vi "Parse NavData.vi"(11 "NavData Port":refnum<k16>) -> (1 "NavData":T1, 3 "NavData Port":refnum<k16>)   [LabVIEW 2011]
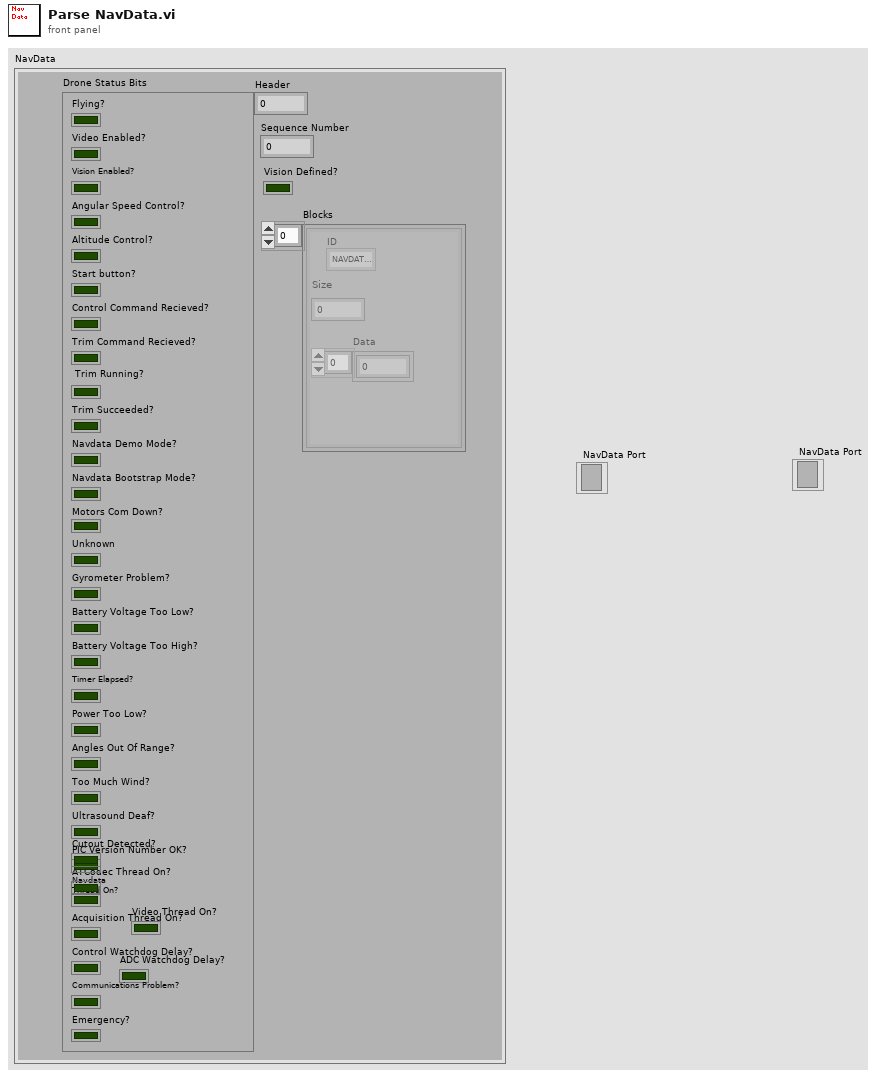
[diagram p1: front panel]
types:
  T1 = cluster{"Drone Status Bits":cluster{"Flying?":bool, "Video Enabled?":bool, "Vision Enabled?":bool, "Angular Speed Control?":bool, "Altitude Control?":bool, "Start button?":bool, "Control Command Recieved?":bool, "Trim Command Recieved?":bool, "Trim Running?":bool, "Trim Succeeded?":bool, "Navdata Demo Mode?":bool, "Navdata Bootstrap Mode?":bool, "Motors Com Down?":bool, "Unknown":bool, "Gyrometer Problem?":bool, "Battery Voltage Too Low?":bool, "Battery Voltage Too High?":bool, "Timer Elapsed?":bool, "Power Too Low?":bool, "Angles Out Of Range?":bool, "Too Much Wind?":bool, "Ultrasound Deaf?":bool, "Cutout Detected?":bool, "PIC Version Number OK?":bool, "ATCodec Thread On?":bool, "Navdata Thread On?":bool, "Video Thread On?":bool, "Acquisition Thread On?":bool, "Control Watchdog Delay?":bool, "ADC Watchdog Delay?":bool, "Communications Problem?":bool, "Emergency?":bool}, "Header":u32, "Sequence Number":u32, "Vision Defined?":bool, "Blocks":cluster{"Size":u16, "Data":u8[], "ID":enum16{"NAVDATA_DEMO", "NAVDATA_TIME", "NAVDATA_RAW_MEASURES", "NAVDATA_PHYS_MEASURES", "NAVDATA_GYROS_OFFSETS", "NAVDATA_EULER_ANGLES", "NAVDATA_REFERENCES", "NAVDATA_TRIMS", "NAVDATA_RC_REFERENCES", "NAVDATA_PWM", "NAVDATA_ALTITUDE", "NAVDATA_VISION_RAW", "NAVDATA_VISION_OF", "NAVDATA_VISION", "NAVDATA_VISION_PERF", "NAVDATA_TRACKERS_SEND", "NAVDATA_VISION_DETECT", "NAVDATA_WATCHDOG", "NAVDATA_ADC_DATA_FRAME", "NAVDATA_VIDEO_STREAM", "NAVDATA_GAMES"}}[]}
  T2 = cluster{"Size":u16, "Data":u8[], "ID":enum16{"NAVDATA_DEMO", "NAVDATA_TIME", "NAVDATA_RAW_MEASURES", "NAVDATA_PHYS_MEASURES", "NAVDATA_GYROS_OFFSETS", "NAVDATA_EULER_ANGLES", "NAVDATA_REFERENCES", "NAVDATA_TRIMS", "NAVDATA_RC_REFERENCES", "NAVDATA_PWM", "NAVDATA_ALTITUDE", "NAVDATA_VISION_RAW", "NAVDATA_VISION_OF", "NAVDATA_VISION", "NAVDATA_VISION_PERF", "NAVDATA_TRACKERS_SEND", "NAVDATA_VISION_DETECT", "NAVDATA_WATCHDOG", "NAVDATA_ADC_DATA_FRAME", "NAVDATA_VIDEO_STREAM", "NAVDATA_GAMES"}}[]
  T3 = cluster{"Size":u16, "Data":u8[], "ID":enum16{"NAVDATA_DEMO", "NAVDATA_TIME", "NAVDATA_RAW_MEASURES", "NAVDATA_PHYS_MEASURES", "NAVDATA_GYROS_OFFSETS", "NAVDATA_EULER_ANGLES", "NAVDATA_REFERENCES", "NAVDATA_TRIMS", "NAVDATA_RC_REFERENCES", "NAVDATA_PWM", "NAVDATA_ALTITUDE", "NAVDATA_VISION_RAW", "NAVDATA_VISION_OF", "NAVDATA_VISION", "NAVDATA_VISION_PERF", "NAVDATA_TRACKERS_SEND", "NAVDATA_VISION_DETECT", "NAVDATA_WATCHDOG", "NAVDATA_ADC_DATA_FRAME", "NAVDATA_VIDEO_STREAM", "NAVDATA_GAMES"}}
  T4 = cluster{"Boolean array[0]":bool, "Boolean array[1]":bool, "Boolean array[2]":bool, "Boolean array[3]":bool, "Boolean array[4]":bool, "Boolean array[5]":bool, "Boolean array[6]":bool, "Boolean array[7]":bool, "Boolean array[8]":bool, "Boolean array[9]":bool, "Boolean array[10]":bool, "Boolean array[11]":bool, "Boolean array[12]":bool, "Boolean array[13]":bool, "Boolean array[14]":bool, "Boolean array[15]":bool, "Boolean array[16]":bool, "Boolean array[17]":bool, "Boolean array[18]":bool, "Boolean array[19]":bool, "Boolean array[20]":bool, "Boolean array[21]":bool, "Boolean array[22]":bool, "Boolean array[23]":bool, "Boolean array[24]":bool, "Boolean array[25]":bool, "Boolean array[26]":bool, "Boolean array[27]":bool, "Boolean array[28]":bool, "Boolean array[29]":bool, "Boolean array[30]":bool, "Boolean array[31]":bool}
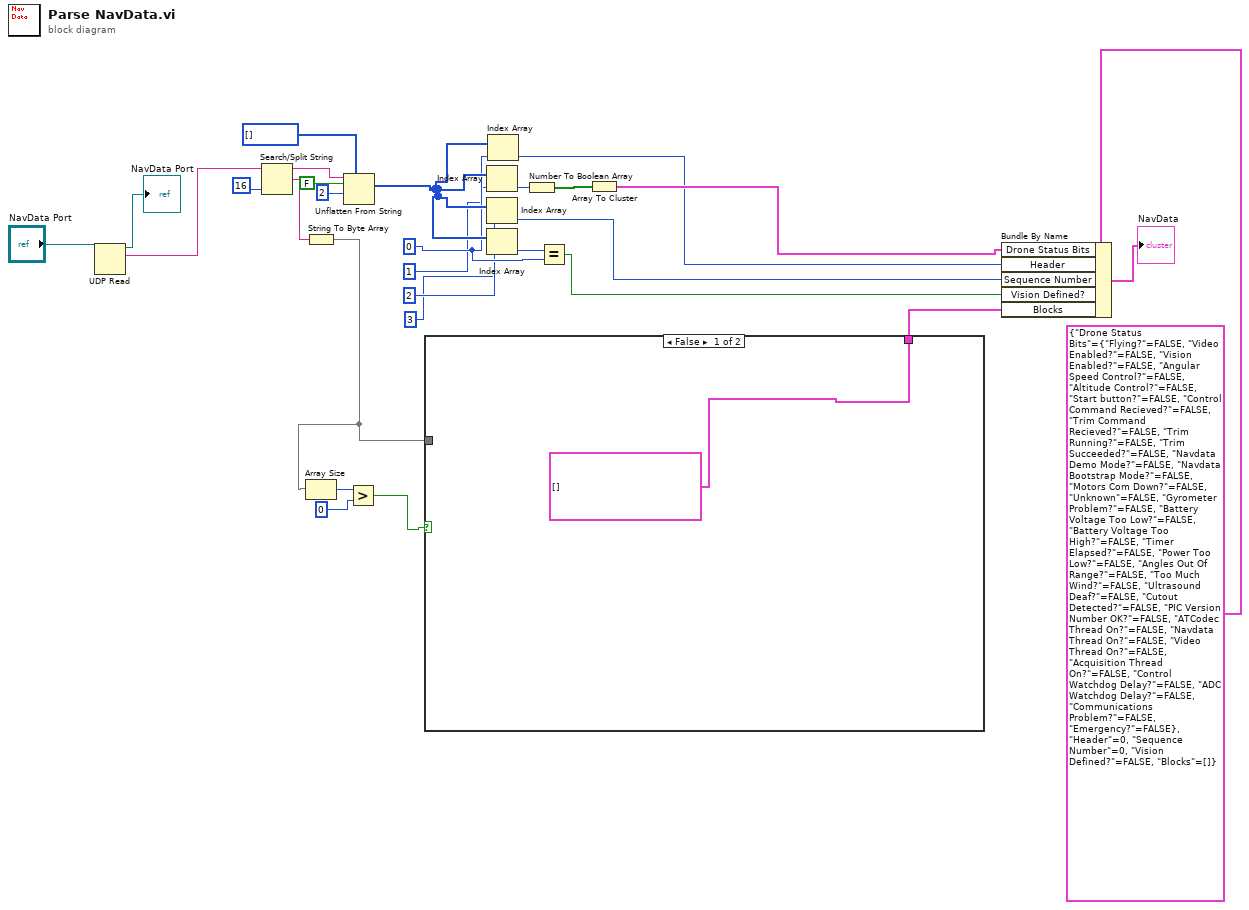
[diagram p0: block diagram]
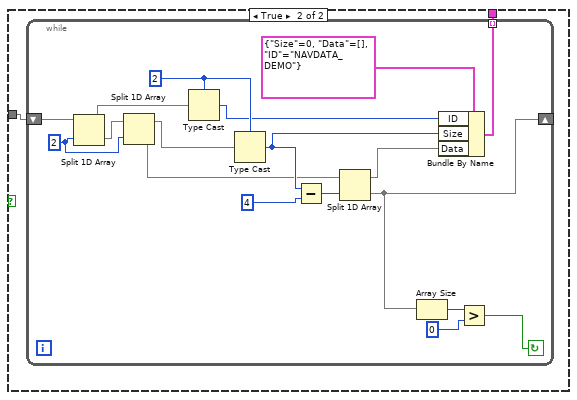
[diagram p2: hidden frame]
diagram:
  w18 = 0
  n1 = UDP Read(connection ID="NavData Port") -> (data out=w2:string, 3:→"NavData Port":refnum<k16>)  [unwired: 3 in, 3 out]
  n2 = Search/Split String(string=w2, offset (0)=16) -> (substring before match=w11:string, match + rest of string=w10:string)  [unwired: 1 in, 1 out]
  n3 = String To Byte Array(string=w10) -> (unsigned byte array=w9:u8[])
  n4 = Array Size(array=w9) -> (size(s)=w8:i32)
  n5 = Unflatten From String(type=u32[] [], binary string=w11, data includes array or string size? (T)=FALSE, byte order (0:big-endian, network order)=u32 2) -> (value=w19:u32[])  [unwired: 1 in, 2 out]
  n6 = Greater?(x=w8, y=0) -> (0:w6:bool)
  n7 = case shown="False" w6 {
    tunnel: w9 -> [_ w31]
    tunnel: [T2 [] ("Blocks") w30] -> w4
    frame False {
    }
    frame True {
      n8 = while {
        shift-right: [w33] -> _
        shift-left: w31 -> [w49]
        tunnel: [w48] -> w30 mode=indexing
        stop <- w34 continue-if-true
        w43 = u16 2
        w46 = 2
        n9 = Split 1D Array(array=w49, index=w46) -> (first subarray=w45:u8[], second subarray=w47:u8[])
        n10 = Split 1D Array(array=w47, index=w46) -> (first subarray=w44:u8[], second subarray=w38:u8[])
        n11 = Type Cast(type=w43, x=w45) -> (*(type *) &x=w42:u16)
        n12 = Type Cast(type=w43, x=w44) -> (*(type *) &x=w40:u16)
        n13 = Subtract(x=w40, y=u16 4) -> (x-y=w41:u16)
        n14 = Split 1D Array(array=w38, index=w41) -> (first subarray=w37:u8[], second subarray=w33:u8[])
        n15 = Array Size(array=w33) -> (size(s)=w36:i32)
        n16 = Bundle By Name(cluster=T3 {"Size"=0, "Data"=[], "ID"=enum."NAVDATA_DEMO"} ("Cluster"), "ID"=w42, "Size"=w40, "Data"=w37) -> (w48:T3)
        n17 = Greater?(x=w36, y=0) -> (0:w34:bool)
      }
    }
  }
  n18 = Index Array(array=w19, index=1) -> (element=w24:u32)
  n19 = Index Array(array=w19, index=2) -> (element=w13:u32)
  n20 = Index Array(array=w19, index=3) -> (element=w23:u32)
  n21 = Index Array(array=w19, index=w18) -> (element=w14:u32)
  n22 = Number To Boolean Array(number=w24) -> (Boolean array=w21:bool[])
  n23 = Equal?(x=w23, y=w18) -> (x = y?=w12:bool)
  n24 = Array To Cluster(array=w21) -> (cluster=w20:T4)
  n25 = Bundle By Name(cluster=T1 {"Drone Status Bits"={"Flying?"=FALSE, "Video Enabled?"=FALSE, "Vision Enabled?"=FALSE, "Angular Speed Control?"=FALSE, "Altitude Control?"=FALSE, "Start button?"=FALSE, "Control Command Recieved?"=FALSE, "Trim Command Recieved?"=FALSE, "Trim Running?"=FALSE, "Trim Succeeded?"=FALSE, "Navdata Demo Mode?"=FALSE, "Navdata Bootstrap Mode?"=FALSE, "Motors Com Down?"=FALSE, "Unknown"=FALSE, "Gyrometer Problem?"=FALSE, "Battery Voltage Too Low?"=FALSE, "Battery Voltage Too High?"=FALSE, "Timer Elapsed?"=FALSE, "Power Too Low?"=FALSE, "Angles Out Of Range?"=FALSE, "Too Much Wind?"=FALSE, "Ultrasound Deaf?"=FALSE, "Cutout Detected?"=FALSE, "PIC Version Number OK?"=FALSE, "ATCodec Thread On?"=FALSE, "Navdata Thread On?"=FALSE, "Video Thread On?"=FALSE, "Acquisition Thread On?"=FALSE, "Control Watchdog Delay?"=FALSE, "ADC Watchdog Delay?"=FALSE, "Communications Problem?"=FALSE, "Emergency?"=FALSE}, "Header"=0, "Sequence Number"=0, "Vision Defined?"=FALSE, "Blocks"=[]} ("NavData"), "Drone Status Bits"=w20, "Header"=w14, "Sequence Number"=w13, "Vision Defined?"=w12, "Blocks"=w4) -> (→"NavData":T1)
